vi "Read Register Map File.vi"(8 "Error In":errorcluster, 11 "RegMap_Name":string="2100_Reg_Map") -> (0 "Error Out":errorcluster, 3 "Main":string[][](array[string]))   [LabVIEW 2013]
uses:
  <vilib>/Utility/file.llb/Read From Spreadsheet File (string).vi
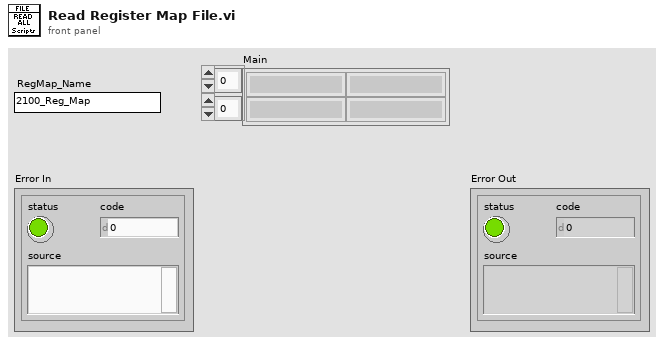
[diagram p1: front panel]
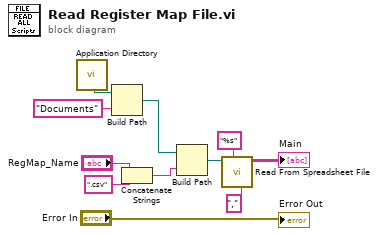
[diagram p0: block diagram]
diagram:
  n1 = call <vilib>:"Application Directory.vi"() -> ("Application Directory"=w3:path)
  n2 = Build Path(base path=w3, name or relative path="Documents") -> (appended path=w1:path)
  n3 = Concatenate Strings("RegMap_Name", ".csv" ("string")) -> (w9:string)
  n4 = Build Path(base path=w1, name or relative path=w9) -> (appended path=w8:path)
  n5 = call-poly <vilib>:"Read From Spreadsheet File.vi"("delimiter (\\t)"="," ("delimiter (\\t)"), "format (%s)"="%s", "file path (dialog if empty)"=w8) -> ("all rows"=→"Main":string[][])  [unwired: 4 in, 4 out]
  "Error Out" <- "Error In"
